vi "Tank_Allowed_Commands.vi"() -> (3 "Array":bool[](array[boolean]))   [LabVIEW 2016]
uses:
  <userlib>/836-libraries/Drive/Drive_Code_V2/Drive_Code_Support/Command_Sends/Drive_Code_Command_List.ctl
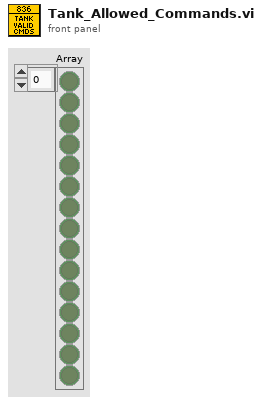
[diagram p1: front panel]
types:
  T1 = typedef "Drive_Code_Command_List.ctl" = enum16{"Do Nothing", "Tank Drive", "Drive Continuous", "Turn", "Drive Distance", "Hold Position", "Hold Yaw", "Follow Camera", "Turn to Camera", "Approach Camera", "PID Update", "Cheesy Drive", "Update Period", "Update PID Inversions"}
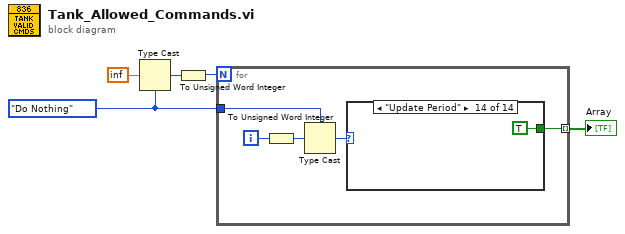
[diagram p0: block diagram]
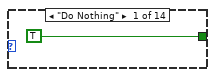
[diagram p2: hidden frame]
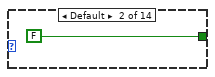
[diagram p3: hidden frame]
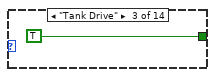
[diagram p4: hidden frame]
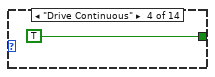
[diagram p5: hidden frame]
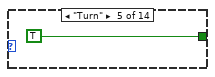
[diagram p6: hidden frame]
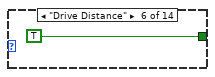
[diagram p7: hidden frame]
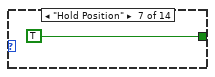
[diagram p8: hidden frame]
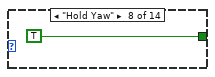
[diagram p9: hidden frame]
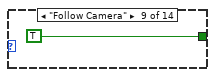
[diagram p10: hidden frame]
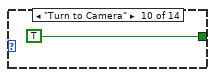
[diagram p11: hidden frame]
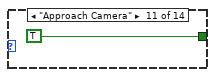
[diagram p12: hidden frame]
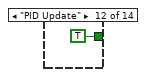
[diagram p13: hidden frame]
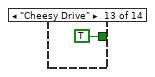
[diagram p14: hidden frame]
diagram:
  w1 = Drive_Code_Command_List."Do Nothing" ("Command")
  n1 = Type Cast(type=w1, x=inf) -> (*(type *) &x=w4:T1)
  n2 = To Unsigned Word Integer(number=w4) -> (unsigned 16bit integer=w3:u16)
  n3 = for {
    N: w3 -> [_]
    tunnel: w1 -> [w9]
    tunnel: [w7] -> w2 mode=indexing
    i -> [w10]
    n4 = To Unsigned Word Integer(number=w10) -> (unsigned 16bit integer=w6:u16)
    n5 = Type Cast(type=w9, x=w6) -> (*(type *) &x=w8:T1)
    n6 = case shown="\"Update Period\"" w8 {
      tunnel: [TRUE FALSE TRUE TRUE TRUE TRUE TRUE TRUE TRUE TRUE TRUE TRUE TRUE TRUE] -> w7
      frame "Do Nothing" {
      }
      frame Default {
      }
      frame "Tank Drive" {
      }
      frame "Drive Continuous" {
      }
      frame "Turn" {
      }
      frame "Drive Distance" {
      }
      frame "Hold Position" {
      }
      frame "Hold Yaw" {
      }
      frame "Follow Camera" {
      }
      frame "Turn to Camera" {
      }
      frame "Approach Camera" {
      }
      frame "PID Update" {
      }
      frame "Cheesy Drive" {
      }
      frame "Update Period" {
      }
    }
  }
  "Array" <- w2
